vi "gRPC Server.vi"(8 "error in (no error)":errorcluster, 11 "CIFTemplatePlugin in":refnum<class "TemplatePlugin.lvclass">) -> (0 "error out":errorcluster, 3 "CIFTemplatePlugin out":refnum<class "TemplatePlugin.lvclass">)   [LabVIEW 2021, in "TemplatePlugin.lvclass"]
uses:
  TemplatePlugin.lvclass
  D:/dev/CIF-LVCore/src/CIFCore/Class/CIFCorePlugin.lvclass
  CIF-LVCore/src/CIFCore/Class/CIFCorePlugin.lvclass/CIFCorePlugin.ctl
  TemplatePlugin.lvclass/TemplatePlugin.ctl
  CIF-LVCore/src/CIFUtilities/CIFOutOfBand/CIFOutOfBand.lvclass/CIFOutOfBand.ctl
  Grpc/Template_server/RPC Messages/cif_template_Status.ctl
  Grpc/Template_server/RPC Messages/cif_template_Result.ctl
  CIF-LVCore/src/CIFCore/Class/Accessors/Read Refresh.vi
  OOB/OOB_Tx/Receive/Read Data.vi
  OOB/OOB_Tx/Receive/Check for OOB Commands.vi
  OOB/OOB_Tx/Private/Read Payload.vi
  CIF-LVCore/src/CIFUtilities/CIFOutOfBand/Read OOB DVR.vi
  OOB/OOB_Tx/Private/Command Settings.vi
  CIF-LVCore/src/CIFUtilities/CIFOutOfBand/Accessors/Read Local OOB Data.vi
  OOB/OOB_Tx/TemplateOOB_Tx.lvclass
  D:/dev/CIF-LVCore/src/CIFUtilities/CIFOutOfBand/CIFOutOfBand.lvclass
  CIF-LVCore/src/CIFCore/Class/CIFCorePlugin.lvclass
  Grpc/Template_server/RPC Service/Template/Template.lvclass
  Grpc/Template_server/Template_server.lvlib
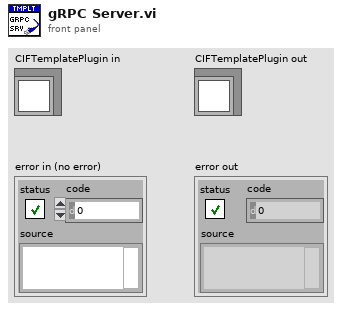
[diagram p1: front panel]
types:
  T1 = typedef "Template_server.lvlib/cif_Template_Status.ctl" = cluster{"code":i32, "message":string}
  T2 = typedef "grpc-lvsupport-release.lvlib/grpcId.ctl" = u64
  T3 = typedef "Template_server.lvlib/cif_Template_Numeric.ctl" = cluster{"numeric":i32}
  T4 = typedef "Template_server.lvlib/cif_Template_Result.ctl" = cluster{"result":i32}
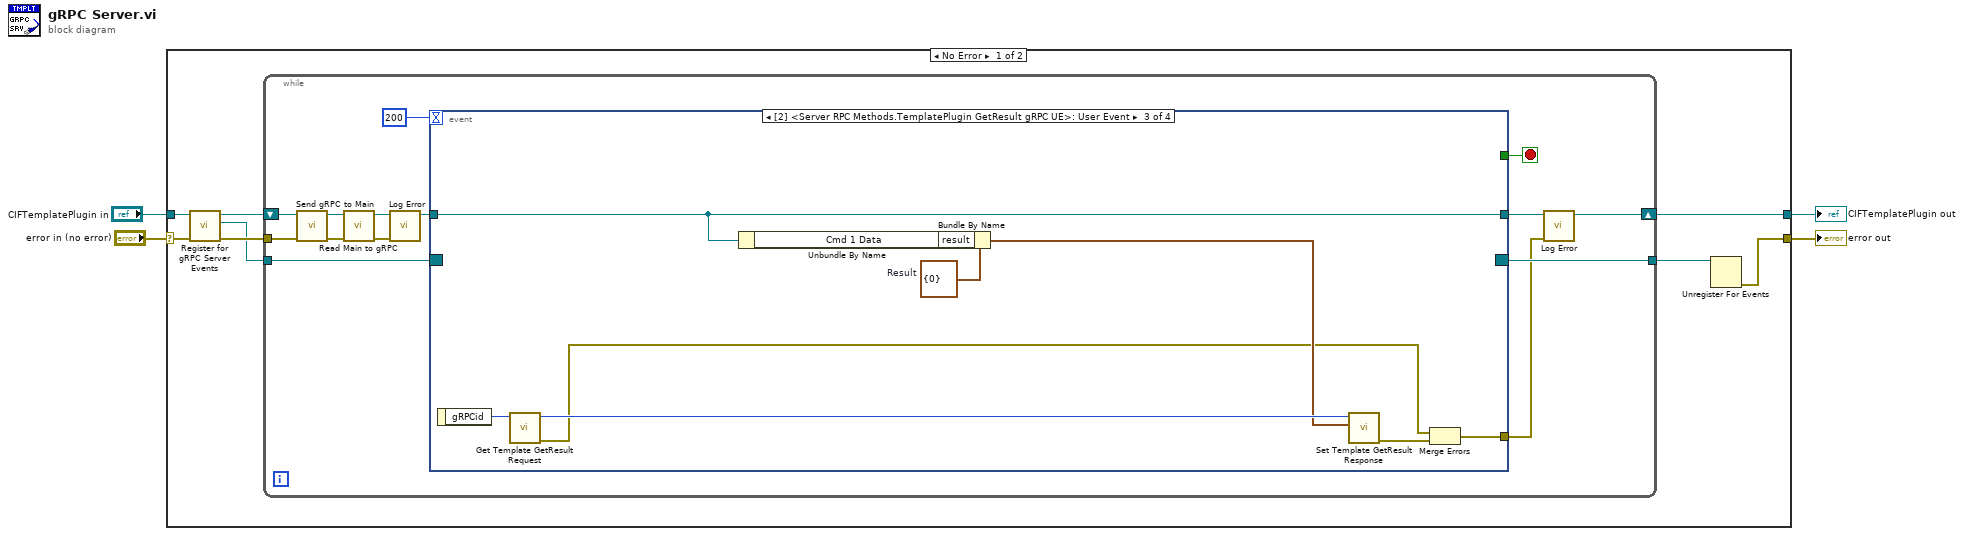
[diagram p0: block diagram]
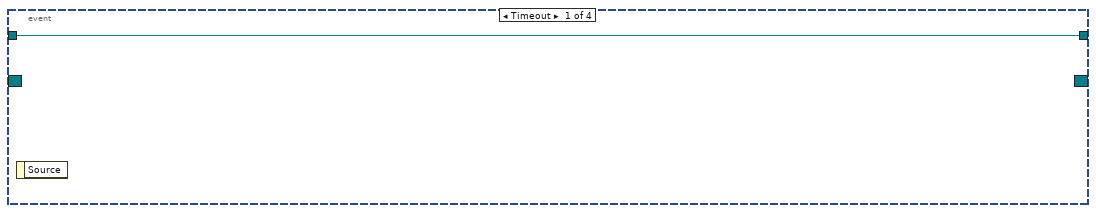
[diagram p2: hidden frame]
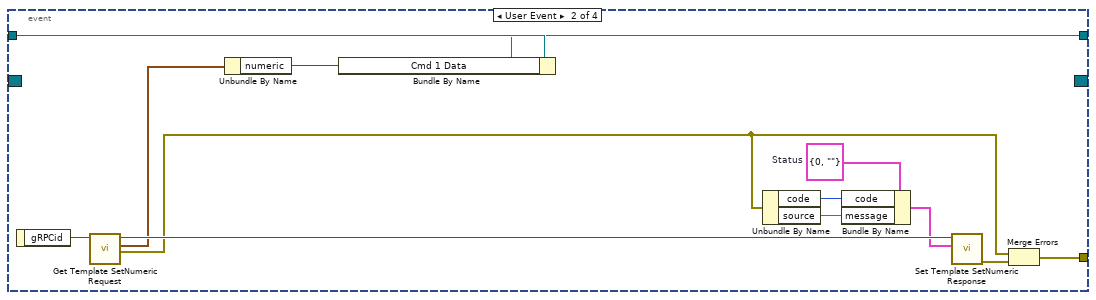
[diagram p3: hidden frame]
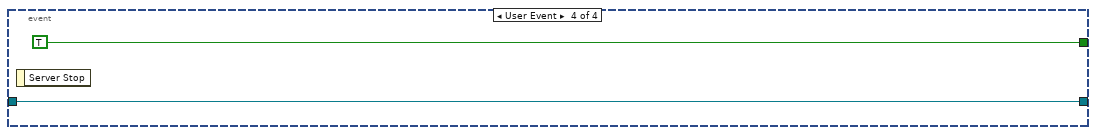
[diagram p4: hidden frame]
diagram:
  n1 = case shown="No Error" "error in (no error)" {
    selector: "error in (no error)" -> [w9 w52]
    tunnel: "CIFTemplatePlugin in" -> [w10 w53]
    tunnel: [w11 w53] -> w2
    tunnel: [w6 w52] -> w1
    frame No Error {
      n2 = call "Register for gRPC Server Events.vi"("error in (no error)"=w9, "CIFTemplatePlugin in"=w10) -> ("error out"=w8:errorcluster, "Event Registration Refnum"=w5:refnum<event-registration>, "CIFTemplatePlugin out"=w7:refnum<class "TemplatePlugin.lvclass">)  [unwired: 7 in]
      n3 = while {
        tunnel: w5 -> [w26]
        tunnel: w8 -> [w17]
        tunnel: [w23] -> w12
        shift-right: [w21] -> w11
        shift-left: w7 -> [w18]
        stop <- w24 stop-if-true
        n4 = call "Send gRPC to Main.vi"("error in (no error)"=w17, "CIFTemplatePlugin in"=w18) -> ("error out"=w15:errorcluster, "CIFTemplatePlugin out"=w16:refnum<class "TemplatePlugin.lvclass">)  [unwired: 8 in]
        n5 = call "Read Main to gRPC.vi"("error in (no error)"=w15, "CIFTemplatePlugin in"=w16) -> ("error out"=w13:errorcluster, "CIFTemplatePlugin out"=w14:refnum<class "TemplatePlugin.lvclass">)  [unwired: 8 in]
        n6 = call "Log Error.vi"("error in (no error)"=w13, "CIFCorePlugin in"=w14) -> ("CIFCorePlugin out"=w19:refnum<class "TemplatePlugin.lvclass">)  [unwired: 8 in, 1 out]
        n7 = event shown="[2] <Server RPC Methods.TemplatePlugin GetResult gRPC UE>: User Event" {
          selector: w26 -> [_ _ _ _]
          dyn-events: [_ _ _ _] -> w23
          timeout: 200 -> [_ _ _ _]
          tunnel: w19 -> [w27 w31 w48 w50]
          tunnel: [_ w38 w49 _] -> w20
          tunnel: [w27 w29 w48 w50] -> w22
          tunnel: [_ _ _ TRUE] -> w24
          event Timeout {
            n8 = event-data() -> ()  [unwired: 1 in, 1 out]
          }
          event User Event {
            w33 = T1 {"code"=0, "message"=""}  # Status
            n9 = event-data() -> ("gRPCid"=w36:T2)  [unwired: 1 in]
            n10 = call "Get Template SetNumeric Request.vi"("gRPCid"=w36) -> ("error out"=w28:errorcluster, "Message Data"=w32:T3, "gRPCid out"=w37:T2)  [unwired: 8 in]
            n11 = Unbundle By Name(w32) -> ("numeric"=w30:i32)
            n12 = Bundle By Name(cluster=w31, "Cmd 1 Data"=w30) -> (w29:refnum<class "TemplatePlugin.lvclass">)
            n13 = Unbundle By Name(w28) -> ("code"=w40:i32, "source"=w39:string)
            n14 = Bundle By Name(cluster=w33, "code"=w40, "message"=w39) -> (w35:T1)
            n15 = call "Set Template SetNumeric Response.vi"("Message Data"=w35, "gRPCid in"=w37) -> ("error out"=w34:errorcluster)  [unwired: 9 in]
            n16 = Merge Errors(w28, w34) -> (w38:errorcluster)
          }
          event User Event {
            w43 = T4 {"result"=0}  # Result
            n17 = event-data() -> ("gRPCid"=w46:T2)  [unwired: 1 in]
            n18 = call "Get Template GetResult Request.vi"("gRPCid"=w46) -> ("error out"=w42:errorcluster, "gRPCid out"=w45:T2)  [unwired: 8 in, 1 out]
            n19 = Unbundle By Name(w48) -> ("Cmd 1 Data"=w47:i32)
            n20 = Bundle By Name(cluster=w43, "result"=w47) -> (w44:T4)
            n21 = call "Set Template GetResult Response.vi"("Message Data"=w44, "gRPCid in"=w45) -> ("error out"=w41:errorcluster)  [unwired: 9 in]
            n22 = Merge Errors(w42, w41) -> (w49:errorcluster)
          }
          event User Event {
            n23 = event-data() -> ()  [unwired: 1 in, 1 out]
          }
        }
        n24 = call "Log Error.vi"("error in (no error)"=w20, "CIFCorePlugin in"=w22) -> ("CIFCorePlugin out"=w21:refnum<class "TemplatePlugin.lvclass">)  [unwired: 8 in, 1 out]
      }
      n25 = Unregister For Events(event registration refnum=w12) -> (error out=w6:errorcluster)  [unwired: 1 in]
    }
    frame Error {
    }
  }
  "error out" <- w1
  "CIFTemplatePlugin out" <- w2
